vi "convert_to_grayscale.vi"(8 "error in (no error)":errorcluster, 11 "Image in":T2) -> (0 "error out":errorcluster, 3 "Image out":T2)   [LabVIEW 2022 SP3, in "Vision.lvlib"]
uses:
  Vision.lvlib
  <vilib>/vision/Image Controls.llb/IMAQ Image.ctl
  bin/Vision.dll
panel:
  in  "Image Type":T1 items=["Grayscale (U8)", "Grayscale (I16)", "Grayscale (SGL)", "Complex (CSG)", "RGB (U32)", "HSL (U32)", "RGB (U64)", "Grayscale (U16)"]
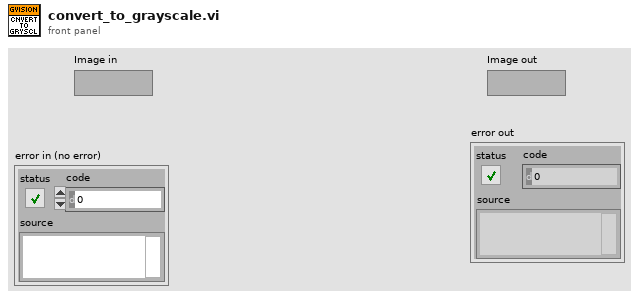
[diagram p1: front panel]
types:
  T1 = typedef "Image Type" = u32
  T2 = typedef "IMAQ Image.ctl" = refnum<image>
  T3 = enum32{"Map Pixel Pointer", "Unmap Pixel Pointer", "Get Pixels Infos"}
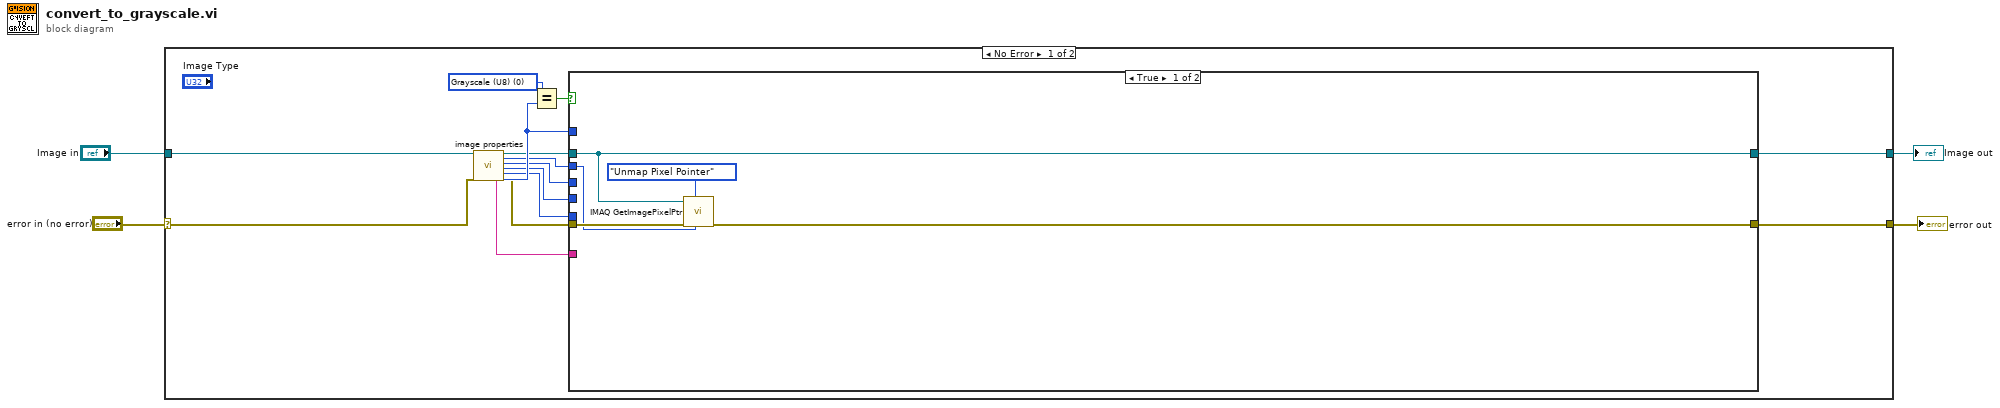
[diagram p0: block diagram]
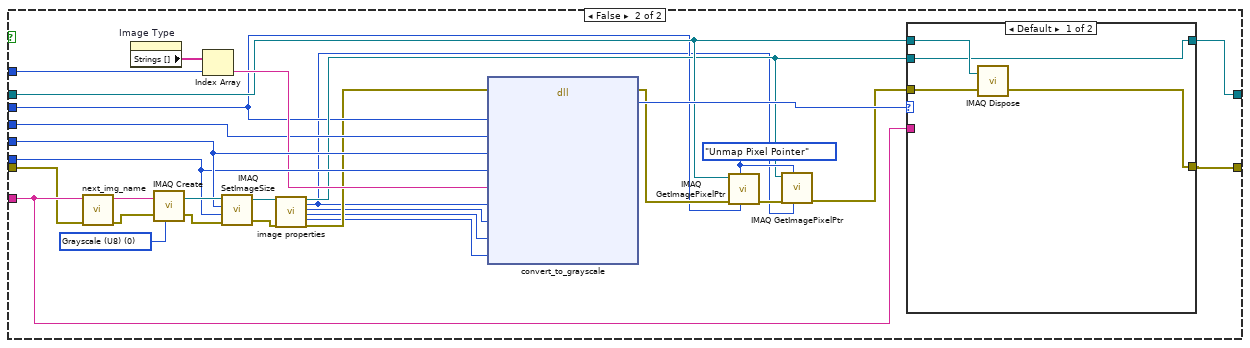
[diagram p2: hidden frame]
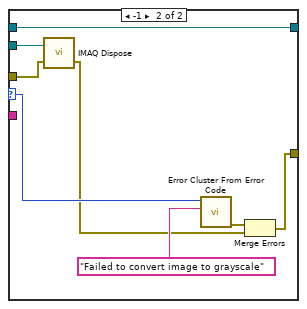
[diagram p3: hidden frame]
diagram:
  n1 = case shown="No Error" "error in (no error)" {
    selector: "error in (no error)" -> [w12 w67]
    tunnel: "Image in" -> [w14 w66]
    tunnel: [w17 w67] -> w2
    tunnel: [w16 w66] -> w1
    frame No Error {
      w15 = T1 0 items=["Grayscale (U8)", "Grayscale (I16)", "Grayscale (SGL)", "Complex (CSG)", "RGB (U32)", "HSL (U32)", "RGB (U64)", "Grayscale (U16)"] ("Image Type")
      n2 = call "image properties.vi"("Image in"=w14, "error in (no error)"=w12) -> ("Image Type"=w13:T1, "Image Name"=w11:string, "Image out"=w7:T2, "Pixel Pointer out"=w6:u64, "Line Width"=w5:i32, "X Resolution"=w10:i32, "Y Resolution"=w9:i32, "error out"=w8:errorcluster)  [unwired: 10 in]
      n3 = Equal?(x=w15, y=w13) -> (x = y?=w18:bool)
      n4 = case shown="True" w18 {
        tunnel: w8 -> [w23 w34]
        tunnel: w7 -> [w19 w39]
        tunnel: [w20 w44] -> w17
        tunnel: [w19 w43] -> w16
        tunnel: w11 -> [_ w36]
        tunnel: w10 -> [_ w50]
        tunnel: w9 -> [_ w49]
        tunnel: w13 -> [_ w47]
        tunnel: w6 -> [w22 w30]
        tunnel: w5 -> [_ w37]
        frame True {
          n5 = call "IMAQ GetImagePixelPtr"("Pixel Pointer in"=w22, "Function"=T3."Unmap Pixel Pointer", "error in (no error)"=w23, "Image"=w19) -> ("error out"=w20:errorcluster)  [unwired: 2 in, 5 out]
        }
        frame False {
          w38 = T3."Unmap Pixel Pointer" ("Function")
          w53 = T1 0 items=["Grayscale (U8)", "Grayscale (I16)", "Grayscale (SGL)", "Complex (CSG)", "RGB (U32)", "HSL (U32)", "RGB (U64)", "Grayscale (U16)"] ("Image Type")
          n6 = call "next_img_name.vi"("error in (no error)"=w34, "name in"=w36) -> ("error out"=w33:errorcluster, "name out"=w35:string)  [unwired: 8 in]
          n7 = property on="Image Type" class="Ring (strict)"() -> ("Strings []"=w48:string[])  [unwired: 2 in, 2 out]
          n8 = call "IMAQ Create"("Image Name"=w35, "Image Type"=w53, "error in (no error)"=w33) -> ("New Image"=w52:T2, "error out"=w51:errorcluster)  [unwired: 2 in]
          n9 = Index Array(array=w48, index=w47) -> (element=w46:string)
          n10 = call "IMAQ SetImageSize"("error in (no error)"=w51, "Y Resolution"=w49, "X Resolution"=w50, "Image"=w52) -> ("error out"=w29:errorcluster, "Image Out"=w32:T2)  [unwired: 1 in]
          n11 = call "image properties.vi"("Image in"=w32, "error in (no error)"=w29) -> ("Image out"=w31:T2, "Pixel Pointer out"=w24:u64, "Line Width"=w27:i32, "X Resolution"=w26:i32, "Y Resolution"=w25:i32, "error out"=w28:errorcluster)  [unwired: 10 in, 2 out]
          n12 = dll-call lib="C:/Users/Caleb/Desktop/nebraska-silicon-lab/pixel-gantry-control/Gantry/Shared Components/bin/Vision.dll" fn="convert_to_grayscale"(error in=w28, "src_imgPtr"=w30, "src_imgLineWidth"=w37, "src_imgWidth"=w50, "src_imgHeight"=w49, "src_type"=w46, "dst_imgPtr"=w24, "dst_imgLineWidth"=w27, "dst_imgWidth"=w26, "dst_imgHeight"=w25) -> (error out=w41:errorcluster, "return type"=w45:i32)  [unwired: 11 in, 1 out]
          n13 = call "IMAQ GetImagePixelPtr"("Pixel Pointer in"=w30, "Function"=w38, "error in (no error)"=w41, "Image"=w39) -> ("error out"=w42:errorcluster)  [unwired: 2 in, 5 out]
          n14 = call "IMAQ GetImagePixelPtr"("Pixel Pointer in"=w24, "Function"=w38, "error in (no error)"=w42, "Image"=w31) -> ("error out"=w40:errorcluster)  [unwired: 2 in, 5 out]
          n15 = case shown="Default" w45 {
            selector: w45 -> [_ w65]
            tunnel: w40 -> [w56 w59]
            tunnel: w31 -> [w55 w60]
            tunnel: [w54 w62] -> w44
            tunnel: w39 -> [w57 w61]
            tunnel: w36 -> [_ _]
            tunnel: [w55 w61] -> w43
            frame Default {
              n16 = call "IMAQ Dispose"("Image"=w57, "error in (no error)"=w56) -> ("error out"=w54:errorcluster)  [unwired: 4 in]
            }
            frame -1 {
              n17 = call "IMAQ Dispose"("Image"=w60, "error in (no error)"=w59) -> ("error out"=w58:errorcluster)  [unwired: 4 in]
              n18 = call <vilib>:"Error Cluster From Error Code.vi"("error message (\"\")"="Failed to convert image to grayscale" ("error message (\"\")"), "error code (0)"=w65) -> ("error out"=w63:errorcluster)  [unwired: 7 in]
              n19 = Merge Errors(w63, w58) -> (w62:errorcluster)
            }
          }
        }
      }
    }
    frame Error {
    }
  }
  "Image out" <- w1
  "error out" <- w2
